vi "IMMU - Convert Gyro.vi"(7 "initialize":bool, 9 "Offset Array In":i16[](array[numeric]), 10 "dt":dbl=1.0 format="%0.2f", 11 "Gyro Data Array In":u8[](array[numeric])) -> (1 "Gyro Rotation Out (degrees)":dbl[](array[numeric]), 3 "Gyro Rotational Velocity Out (deg/s)":dbl[](array[numeric]))   [LabVIEW 2021]
uses:
  <vilib>/ptbypt/NI_PtbyPt.lvlib
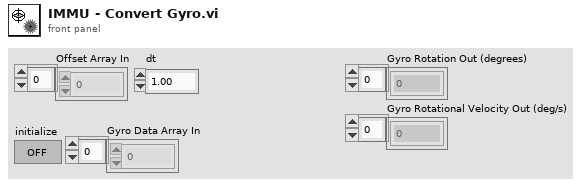
[diagram p1: front panel]
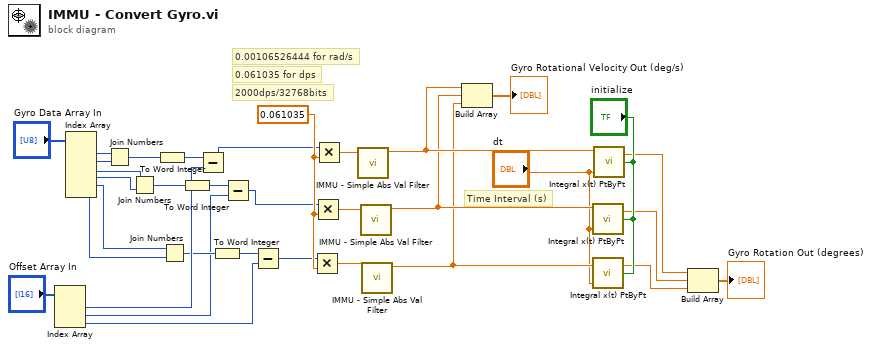
[diagram p0: block diagram]
diagram:
  w12 = 0.061035 ("y")
  # "0.00106526444 for rad/s"
  # "0.061035 for dps"
  # "2000dps/32768bits"
  # "Time Interval (s)"
  n1 = Index Array(array="Offset Array In") -> (element #1=w32:i16, element #2=w17:i16, element #3=w18:i16)  [unwired: 3 in]
  n2 = Index Array(array="Gyro Data Array In") -> (element #1=w29:u8, element #2=w28:u8, element #3=w15:u8, element #4=w16:u8, element #5=w14:u8, element #6=w13:u8)  [unwired: 6 in]
  n3 = Join Numbers(hi=w29, lo=w28) -> ((hi.lo)=w34:u16)
  n4 = Join Numbers(hi=w15, lo=w16) -> ((hi.lo)=w22:u16)
  n5 = To Word Integer(number=w34) -> (16bit integer=w33:i16)
  n6 = Join Numbers(hi=w14, lo=w13) -> ((hi.lo)=w20:u16)
  n7 = To Word Integer(number=w22) -> (16bit integer=w21:i16)
  n8 = Subtract(x=w33, y=w32) -> (x-y=w11:i16)
  n9 = To Word Integer(number=w20) -> (16bit integer=w19:i16)
  n10 = Subtract(x=w21, y=w17) -> (x-y=w10:i16)
  n11 = Subtract(x=w19, y=w18) -> (x-y=w9:i16)
  n12 = Multiply(x=w9, y=w12) -> (x*y=w7:dbl)
  n13 = Multiply(x=w10, y=w12) -> (x*y=w6:dbl)
  n14 = Multiply(x=w11, y=w12) -> (x*y=w8:dbl)
  n15 = call "IMMU - Simple Abs Val Filter.vi"("Value In"=w8) -> ("Output"=w5:dbl)  [unwired: 10 in]
  n16 = call "IMMU - Simple Abs Val Filter.vi"("Value In"=w6) -> ("Output"=w4:dbl)  [unwired: 10 in]
  n17 = call "IMMU - Simple Abs Val Filter.vi"("Value In"=w7) -> ("Output"=w3:dbl)  [unwired: 10 in]
  n18 = Build Array(w5, w4, w3) -> (→"Gyro Rotational Velocity Out (deg/s)":dbl[])
  n19 = call <vilib>:"Integral x(t) PtByPt.vi"("initialize"="initialize", "dt"="dt", "x"=w4) -> ("integral x(t)"=w25:dbl)  [unwired: 1 in, 1 out]
  n20 = call <vilib>:"Integral x(t) PtByPt.vi"("initialize"="initialize", "dt"="dt", "x"=w3) -> ("integral x(t)"=w24:dbl)  [unwired: 1 in, 1 out]
  n21 = call <vilib>:"Integral x(t) PtByPt.vi"("initialize"="initialize", "dt"="dt", "x"=w5) -> ("integral x(t)"=w26:dbl)  [unwired: 1 in, 1 out]
  n22 = Build Array(w26, w25, w24) -> (→"Gyro Rotation Out (degrees)":dbl[])
